vi "Get BLISS_Next Server or Done.vi"(7 "Queue in":refnum<queue>, 8 "error in":errorcluster, 11 "Data Parameters in":T1={"Server Index"=0, "username"="", "password"="", "Server Status List"=[{"Server Name"="BlissUT124", "connection\nsuccessful"=TRUE}, {"Server Name"="BlissMP146", "connection\nsuccessful"=TRUE}, {"Server Name"="BlissMP145", "connection\nsuccessful"=TRUE}, {"Server Name"="BlissMP140", "connection\nsuccessful"=TRUE}, {"Server Name"="BlissMP137", "connection\nsuccessful"=TRUE}, {"Server Name"="BlissMP135", "connection\nsuccessful"=TRUE}, {"Server Name"="BlissMP134", "connection\nsuccessful"=TRUE}, {"Server Name"="BlissMP132", "connection\nsuccessful"=TRUE}, {"Server Name"="BlissMA109", "connection\nsuccessful"=TRUE}, {"Server Name"="BlissMA107", "connection\nsuccessful"=TRUE}, {"Server Name"="BlissMA106", "connection\nsuccessful"=TRUE}, {"Server Name"="BlissMA101", "connection\nsuccessful"=TRUE}, {"Server Name"="BlissLU118", "connection\nsuccessful"=TRUE}, {"Server Name"="BlissLU117", "connection\nsuccessful"=TRUE}, {"Server Name"="BlissLU116", "connection\nsuccessful"=TRUE}, {"Server Name"="BlissLU115", "connection\nsuccessful"=TRUE}, {"Server Name"="BlissLU114", "connection\nsuccessful"=TRUE}, {"Server Name"="BlissLU113", "connection\nsuccessful"=TRUE}, {"Server Name"="BlissLU111", "connection\nsuccessful"=TRUE}, {"Server Name"="BlissLL185", "connection\nsuccessful"=TRUE}, {"Server Name"="BlissLL183", "connection\nsuccessful"=TRUE}, {"Server Name"="BlissLL173", "connection\nsuccessful"=TRUE}, {"Server Name"="BlissLL172", "connection\nsuccessful"=TRUE}, {"Server Name"="BlissLL171", "connection\nsuccessful"=TRUE}, {"Server Name"="BlissJH103", "connection\nsuccessful"=TRUE}, {"Server Name"="BlissJH102", "connection\nsuccessful"=TRUE}, {"Server Name"="BlissJH101", "connection\nsuccessful"=TRUE}, {"Server Name"="BlissJE116", "connection\nsuccessful"=TRUE}, {"Server Name"="BlissJE115", "connection\nsuccessful"=TRUE}, {"Server Name"="BlissJE114", "connection\nsuccessful"=TRUE}, {"Server Name"="BlissJE111", "connection\nsuccessful"=TRUE}, {"Server Name"="BlissHD183", "connection\nsuccessful"=TRUE}, {"Server Name"="BlissHD182", "connection\nsuccessful"=TRUE}, {"Server Name"="BlissHD181", "connection\nsuccessful"=TRUE}, {"Server Name"="BlissGPDFFPL", "connection\nsuccessful"=TRUE}, {"Server Name"="BlissEUWIPES", "connection\nsuccessful"=TRUE}, {"Server Name"="BlissEU179", "connection\nsuccessful"=TRUE}, {"Server Name"="BlissEU178", "connection\nsuccessful"=TRUE}, {"Server Name"="BlissEU177", "connection\nsuccessful"=TRUE}, {"Server Name"="Blissdvds02", "connection\nsuccessful"=TRUE}, {"Server Name"="BlissDOWIPES", "connection\nsuccessful"=TRUE}, {"Server Name"="BlissCR022", "connection\nsuccessful"=TRUE}, {"Server Name"="BlissCR021", "connection\nsuccessful"=TRUE}, {"Server Name"="BlissCG167", "connection\nsuccessful"=TRUE}, {"Server Name"="BlissCG166", "connection\nsuccessful"=TRUE}, {"Server Name"="BlissCG161", "connection\nsuccessful"=TRUE}, {"Server Name"="BlissCG160", "connection\nsuccessful"=TRUE}, {"Server Name"="BlissCG159", "connection\nsuccessful"=TRUE}, {"Server Name"="BlissCG158", "connection\nsuccessful"=TRUE}, {"Server Name"="BlissCG157", "connection\nsuccessful"=TRUE}, {"Server Name"="BlissCG156", "connection\nsuccessful"=TRUE}, {"Server Name"="BlissCG151", "connection\nsuccessful"=TRUE}, {"Server Name"="BlissCB172", "connection\nsuccessful"=TRUE}, {"Server Name"="BlissCB171", "connection\nsuccessful"=TRUE}, {"Server Name"="BlissCB108", "connection\nsuccessful"=TRUE}, {"Server Name"="BlissCB107", "connection\nsuccessful"=TRUE}, {"Server Name"="BlissBV181", "connection\nsuccessful"=TRUE}, {"Server Name"="BlissBV162", "connection\nsuccessful"=TRUE}, {"Server Name"="BlissAK177", "connection\nsuccessful"=TRUE}, {"Server Name"="BlissAK176", "connection\nsuccessful"=TRUE}, {"Server Name"="BlissAK175", "connection\nsuccessful"=TRUE}, {"Server Name"="BlissAK174", "connection\nsuccessful"=TRUE}, {"Server Name"="BlissAK173", "connection\nsuccessful"=TRUE}, {"Server Name"="BlissAK172", "connection\nsuccessful"=TRUE}, {"Server Name"="BlissAK171", "connection\nsuccessful"=TRUE}, {"Server Name"="BlissAK139", "connection\nsuccessful"=TRUE}, {"Server Name"="BlissAK134", "connection\nsuccessful"=TRUE}, {"Server Name"="BlissAK131", "connection\nsuccessful"=TRUE}, {"Server Name"="BlissAH163", "connection\nsuccessful"=TRUE}, {"Server Name"="BlissAH162", "connection\nsuccessful"=TRUE}, {"Server Name"="BlissAH161", "connection\nsuccessful"=TRUE}, {"Server Name"="BlissAH122", "connection\nsuccessful"=TRUE}, {"Server Name"="BlissAH121", "connection\nsuccessful"=TRUE}, {"Server Name"="BlissAD106", "connection\nsuccessful"=TRUE}, {"Server Name"="BlissAD104", "connection\nsuccessful"=TRUE}, {"Server Name"="BlissAB105", "connection\nsuccessful"=TRUE}, {"Server Name"="BlissAB104", "connection\nsuccessful"=TRUE}], "search criteria"={"views"="*.", "reject codes"="*.", "sizes"="*.", "BLISS Image Types"=enum."Get Both PBQA And Reject Images", "Start Timestamp"=timestamp(2145895200 s since 1904-01-01), "End Timesteamp"=timestamp(34618039200 s since 1904-01-01), "# Images per folder"=1, "Reset Filters Button"=FALSE}, "PBQA File List"=[], "Reject File List"=[], "Save to Folder"=path "", "Server List"=["BlissAB102", "BlissAB103", "BlissAB104", "BlissAB105", "BlissAD104", "BlissAD106", "BlissAH111", "BlissAH112", "BlissAH114", "BlissAH121", "BlissAH122", "BlissAH161", "BlissAH162", "BlissAH163", "BlissAK131", "BlissAK134", "BlissAK139", "BlissAK171", "BlissAK172", "BlissAK173", "BlissAK174", "BlissAK175", "BlissAK176", "BlissAK177", "BlissBH110", "BlissBV162", "BlissBV181", "BlissCB107", "BlissCB108", "BlissCB171", "BlissCB172", "BlissCG151", "BlissCG156", "BlissCG157", "BlissCG158", "BlissCG159", "BlissCG160", "BlissCG161", "BlissCG166", "BlissCG167", "BlissCR013", "BlissCR015", "BlissCR016", "BlissCR020", "BlissCR021", "BlissCR022", "BlissCR119", "BlissCRDev01", "BlissDOWIPES", "Blissdvds02", "BlissEU135D", "BlissEU177", "BlissEU178", "BlissEU179", "BlissEUDS001", "BlissEUWIPES", "BlissGPDFFPL", "BlissHD181", "BlissHD182", "BlissHD183", "BlissJE111", "BlissJE112", "BlissJE114", "BlissJE115", "BlissJE116", "BlissJH101", "BlissJH102", "BlissJH103", "BlissLL171", "BlissLL172", "BlissLL173", "BlissLL174", "BlissLL183", "BlissLL185", "BlissLS101", "BlissLS102", "BlissLU111", "BlissLU113", "BlissLU114", "BlissLU115", "BlissLU116", "BlissLU117", "BlissLU118", "BlissMA101", "BlissMA106", "BlissMA107", "BlissMA109", "BlissMP132", "BlissMP133", "BlissMP134", "BlissMP135", "BlissMP136", "BlissMP137", "BlissMP138", "BlissMP140", "BlissMP145", "BlissMP146", "BlissMP147", "BlissMR111", "BlissMR112", "BlissMR113", "BlissMX101", "BlissMX171", "BlissMX172", "BlissMX173", "BlissMX174", "BlissMX175", "BlissMX176", "BlissMX177", "BlissNK101", "BlissNK104", "BlissNK105", "BlissNK106", "BlissNK107", "BlissOC101", "BlissOC102", "BlissOC103", "BlissOC104", "BlissOC109", "BlissOC110", "BlissPESDXL", "BlissSI110", "BlissTR005", "BlissTR101", "BlissTR104", "BlissTR106", "BlissTR109", "BlissTR110", "BlissTR111", "BlissTR112", "BlissTR113", "BlissTR114", "BlissTR115", "BlissTR116", "BlissUT122", "BlissUT123", "BlissUT124", "BlissVP101", "BlissVP171"], "Start Time"=timestamp(3690155740.033191 s since 1904-01-01), "Use Line Subfolders"=FALSE, "Use View Subfolders"=FALSE} {"search criteria"."# Images per folder" min=1 max=10 step=1}) -> (0 "error out":errorcluster, 3 "Data Parameters out":T1={"Server Index"=138, "username"="varga.sm@pg.com", "password"="Magyar09", "Server Status List"=[{"Server Name"="BlissUT124", "connection\nsuccessful"=TRUE}, {"Server Name"="BlissMP146", "connection\nsuccessful"=TRUE}, {"Server Name"="BlissMP145", "connection\nsuccessful"=TRUE}, {"Server Name"="BlissMP140", "connection\nsuccessful"=TRUE}, {"Server Name"="BlissMP137", "connection\nsuccessful"=TRUE}, {"Server Name"="BlissMP135", "connection\nsuccessful"=TRUE}, {"Server Name"="BlissMP134", "connection\nsuccessful"=TRUE}, {"Server Name"="BlissMP132", "connection\nsuccessful"=TRUE}, {"Server Name"="BlissMA109", "connection\nsuccessful"=TRUE}, {"Server Name"="BlissMA107", "connection\nsuccessful"=TRUE}, {"Server Name"="BlissMA106", "connection\nsuccessful"=TRUE}, {"Server Name"="BlissMA101", "connection\nsuccessful"=TRUE}, {"Server Name"="BlissLU118", "connection\nsuccessful"=TRUE}, {"Server Name"="BlissLU117", "connection\nsuccessful"=TRUE}, {"Server Name"="BlissLU116", "connection\nsuccessful"=TRUE}, {"Server Name"="BlissLU115", "connection\nsuccessful"=TRUE}, {"Server Name"="BlissLU114", "connection\nsuccessful"=TRUE}, {"Server Name"="BlissLU113", "connection\nsuccessful"=TRUE}, {"Server Name"="BlissLU111", "connection\nsuccessful"=TRUE}, {"Server Name"="BlissLL185", "connection\nsuccessful"=TRUE}, {"Server Name"="BlissLL183", "connection\nsuccessful"=TRUE}, {"Server Name"="BlissLL173", "connection\nsuccessful"=TRUE}, {"Server Name"="BlissLL172", "connection\nsuccessful"=TRUE}, {"Server Name"="BlissLL171", "connection\nsuccessful"=TRUE}, {"Server Name"="BlissJH103", "connection\nsuccessful"=TRUE}, {"Server Name"="BlissJH102", "connection\nsuccessful"=TRUE}, {"Server Name"="BlissJH101", "connection\nsuccessful"=TRUE}, {"Server Name"="BlissJE116", "connection\nsuccessful"=TRUE}, {"Server Name"="BlissJE115", "connection\nsuccessful"=TRUE}, {"Server Name"="BlissJE114", "connection\nsuccessful"=TRUE}, {"Server Name"="BlissJE111", "connection\nsuccessful"=TRUE}, {"Server Name"="BlissHD183", "connection\nsuccessful"=TRUE}, {"Server Name"="BlissHD182", "connection\nsuccessful"=TRUE}, {"Server Name"="BlissHD181", "connection\nsuccessful"=TRUE}, {"Server Name"="BlissGPDFFPL", "connection\nsuccessful"=TRUE}, {"Server Name"="BlissEUWIPES", "connection\nsuccessful"=TRUE}, {"Server Name"="BlissEU179", "connection\nsuccessful"=TRUE}, {"Server Name"="BlissEU178", "connection\nsuccessful"=TRUE}, {"Server Name"="BlissEU177", "connection\nsuccessful"=TRUE}, {"Server Name"="Blissdvds02", "connection\nsuccessful"=TRUE}, {"Server Name"="BlissDOWIPES", "connection\nsuccessful"=TRUE}, {"Server Name"="BlissCR022", "connection\nsuccessful"=TRUE}, {"Server Name"="BlissCR021", "connection\nsuccessful"=TRUE}, {"Server Name"="BlissCG167", "connection\nsuccessful"=TRUE}, {"Server Name"="BlissCG166", "connection\nsuccessful"=TRUE}, {"Server Name"="BlissCG161", "connection\nsuccessful"=TRUE}, {"Server Name"="BlissCG160", "connection\nsuccessful"=TRUE}, {"Server Name"="BlissCG159", "connection\nsuccessful"=TRUE}, {"Server Name"="BlissCG158", "connection\nsuccessful"=TRUE}, {"Server Name"="BlissCG157", "connection\nsuccessful"=TRUE}, {"Server Name"="BlissCG156", "connection\nsuccessful"=TRUE}, {"Server Name"="BlissCG151", "connection\nsuccessful"=TRUE}, {"Server Name"="BlissCB172", "connection\nsuccessful"=TRUE}, {"Server Name"="BlissCB171", "connection\nsuccessful"=TRUE}, {"Server Name"="BlissCB108", "connection\nsuccessful"=TRUE}, {"Server Name"="BlissCB107", "connection\nsuccessful"=TRUE}, {"Server Name"="BlissBV181", "connection\nsuccessful"=TRUE}, {"Server Name"="BlissBV162", "connection\nsuccessful"=TRUE}, {"Server Name"="BlissAK177", "connection\nsuccessful"=TRUE}, {"Server Name"="BlissAK176", "connection\nsuccessful"=TRUE}, {"Server Name"="BlissAK175", "connection\nsuccessful"=TRUE}, {"Server Name"="BlissAK174", "connection\nsuccessful"=TRUE}, {"Server Name"="BlissAK173", "connection\nsuccessful"=TRUE}, {"Server Name"="BlissAK172", "connection\nsuccessful"=TRUE}, {"Server Name"="BlissAK171", "connection\nsuccessful"=TRUE}, {"Server Name"="BlissAK139", "connection\nsuccessful"=TRUE}, {"Server Name"="BlissAK134", "connection\nsuccessful"=TRUE}, {"Server Name"="BlissAK131", "connection\nsuccessful"=TRUE}, {"Server Name"="BlissAH163", "connection\nsuccessful"=TRUE}, {"Server Name"="BlissAH162", "connection\nsuccessful"=TRUE}, {"Server Name"="BlissAH161", "connection\nsuccessful"=TRUE}, {"Server Name"="BlissAH122", "connection\nsuccessful"=TRUE}, {"Server Name"="BlissAH121", "connection\nsuccessful"=TRUE}, {"Server Name"="BlissAD106", "connection\nsuccessful"=TRUE}, {"Server Name"="BlissAD104", "connection\nsuccessful"=TRUE}, {"Server Name"="BlissAB105", "connection\nsuccessful"=TRUE}, {"Server Name"="BlissAB104", "connection\nsuccessful"=TRUE}], "search criteria"={"views"="VISFE1,VISCC2", "reject codes"="R325,R326", "sizes"="S2,S3,S4,S5,S6,S7", "BLISS Image Types"=enum."Get Only Reject Images", "Start Timestamp"=timestamp(2145895200 s since 1904-01-01), "End Timesteamp"=timestamp(34618039200 s since 1904-01-01), "# Images per folder"=1, "Reset Filters Button"=FALSE}, "PBQA File List"=[], "Reject File List"=[], "Save to Folder"=path "D:/One Drive PG/Procter and Gamble/Varghese, Jacob - Deep Learning Vision System/Front Ear Foldover/BLISS Rejects (only R325 + R326) - not reviewed", "Server List"=["BlissAB102", "BlissAB103", "BlissAB104", "BlissAB105", "BlissAD104", "BlissAD106", "BlissAH111", "BlissAH112", "BlissAH114", "BlissAH121", "BlissAH122", "BlissAH161", "BlissAH162", "BlissAH163", "BlissAK131", "BlissAK134", "BlissAK139", "BlissAK171", "BlissAK172", "BlissAK173", "BlissAK174", "BlissAK175", "BlissAK176", "BlissAK177", "BlissBH110", "BlissBV162", "BlissBV181", "BlissCB107", "BlissCB108", "BlissCB171", "BlissCB172", "BlissCG151", "BlissCG156", "BlissCG157", "BlissCG158", "BlissCG159", "BlissCG160", "BlissCG161", "BlissCG166", "BlissCG167", "BlissCR013", "BlissCR015", "BlissCR016", "BlissCR020", "BlissCR021", "BlissCR022", "BlissCR119", "BlissCRDev01", "BlissDOWIPES", "Blissdvds02", "BlissEU135D", "BlissEU177", "BlissEU178", "BlissEU179", "BlissEUDS001", "BlissEUWIPES", "BlissGPDFFPL", "BlissHD181", "BlissHD182", "BlissHD183", "BlissJE111", "BlissJE112", "BlissJE114", "BlissJE115", "BlissJE116", "BlissJH101", "BlissJH102", "BlissJH103", "BlissLL171", "BlissLL172", "BlissLL173", "BlissLL174", "BlissLL183", "BlissLL185", "BlissLS101", "BlissLS102", "BlissLU111", "BlissLU113", "BlissLU114", "BlissLU115", "BlissLU116", "BlissLU117", "BlissLU118", "BlissMA101", "BlissMA106", "BlissMA107", "BlissMA109", "BlissMP132", "BlissMP133", "BlissMP134", "BlissMP135", "BlissMP136", "BlissMP137", "BlissMP138", "BlissMP140", "BlissMP145", "BlissMP146", "BlissMP147", "BlissMR111", "BlissMR112", "BlissMR113", "BlissMX101", "BlissMX171", "BlissMX172", "BlissMX173", "BlissMX174", "BlissMX175", "BlissMX176", "BlissMX177", "BlissNK101", "BlissNK104", "BlissNK105", "BlissNK106", "BlissNK107", "BlissOC101", "BlissOC102", "BlissOC103", "BlissOC104", "BlissOC109", "BlissOC110", "BlissPESDXL", "BlissSI110", "BlissTR005", "BlissTR101", "BlissTR104", "BlissTR106", "BlissTR109", "BlissTR110", "BlissTR111", "BlissTR112", "BlissTR113", "BlissTR114", "BlissTR115", "BlissTR116", "BlissUT122", "BlissUT123", "BlissUT124", "BlissVP101", "BlissVP171"], "Start Time"=timestamp(3690155740.033191 s since 1904-01-01), "Use Line Subfolders"=FALSE, "Use View Subfolders"=FALSE} {"search criteria"."# Images per folder" min=1 max=10 step=1})   [LabVIEW 2020]
uses:
  Get BLISS_Data Paramter Actions.ctl
  MC5e Gobal_Variables.vi
  Get BLISS_Global Command Q Control.ctl
  MC5e Squad_Info.ctl
  MC5e Unit_Status_List.ctl
  Get BLISS_Search Criteria.ctl
  MC5e Data_Parameters.ctl
panel:
  # "Reject codes only apply to rejects"
  # "Size filters only apply to PBQA folders"
  # "Reject codes only apply to rejects"
  # "Size filters only apply to PBQA folders"
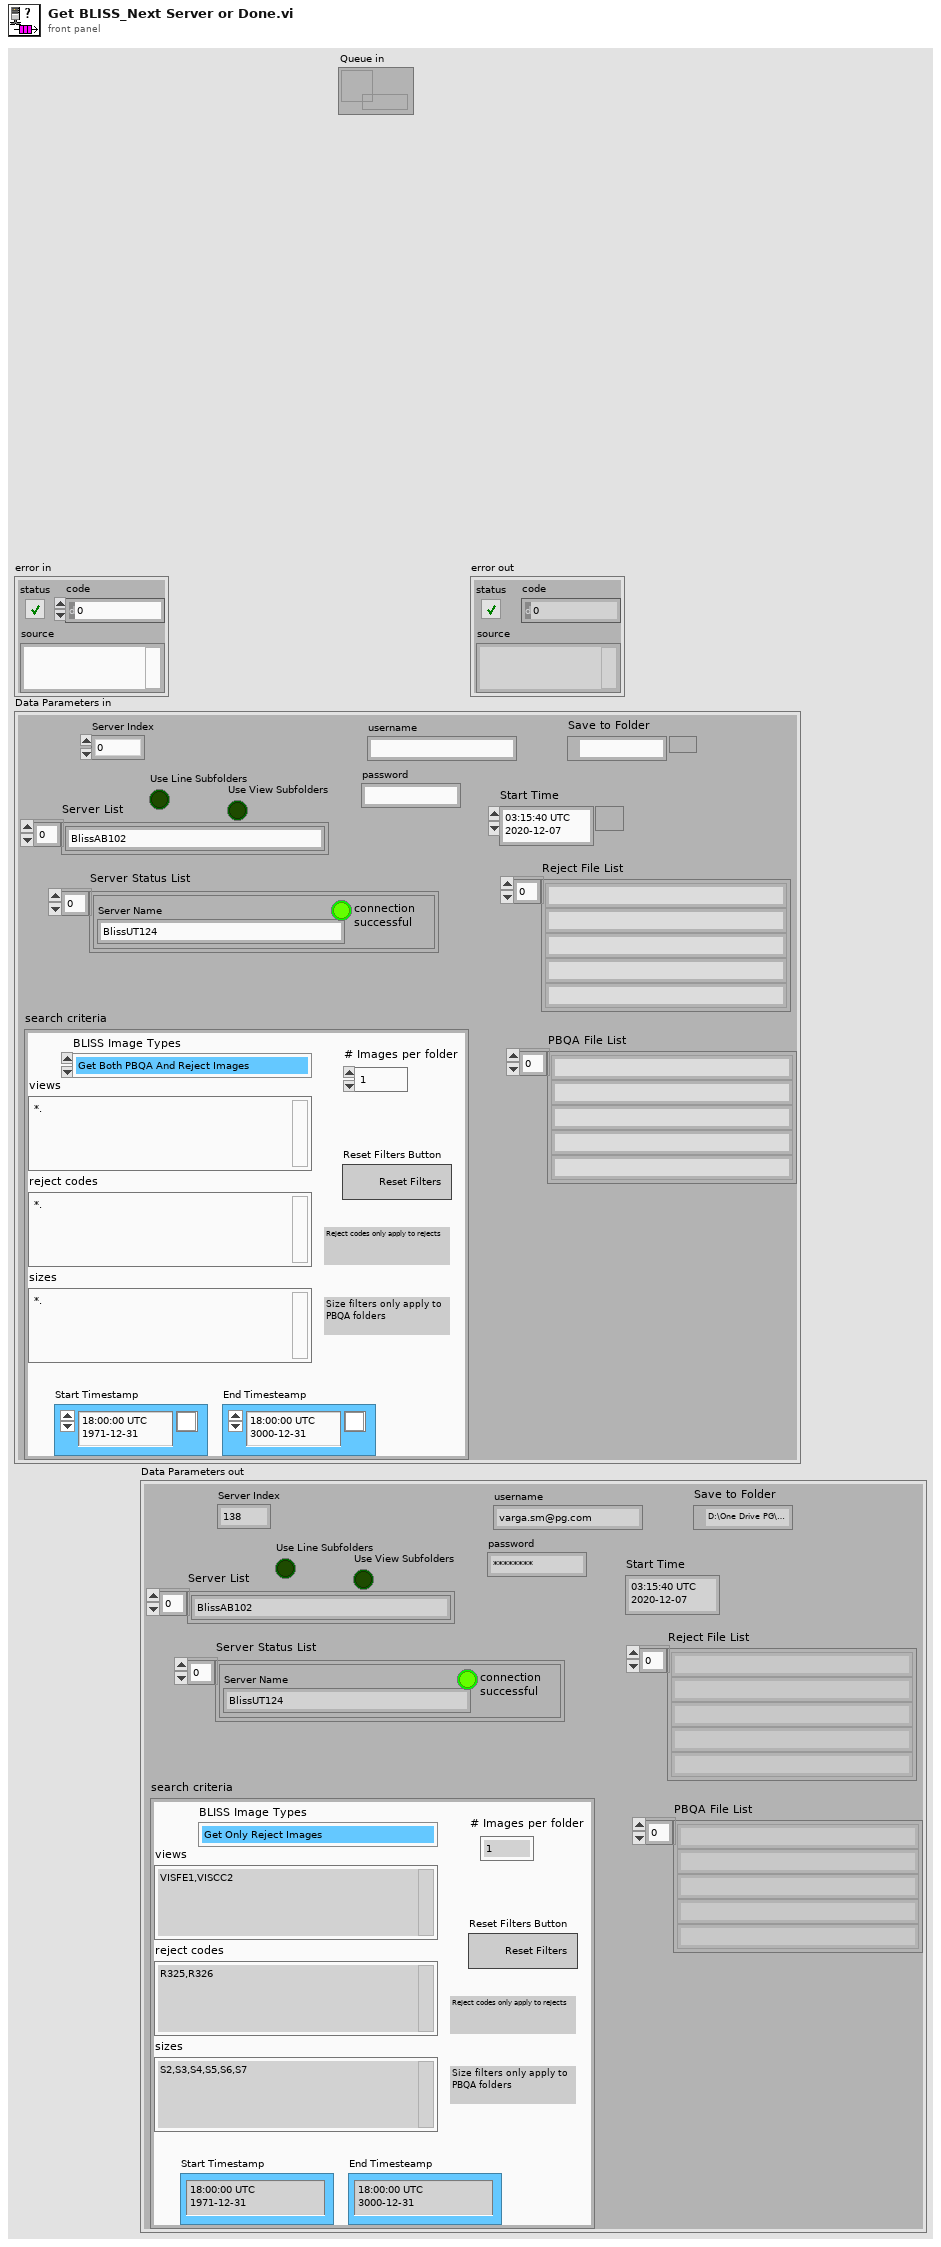
[diagram p1: front panel]
types:
  T1 = typedef "MC5e Data_Parameters.ctl" = cluster{"Server Index":i32, "username":string, "password":string, "Server Status List":T2, "search criteria":T4, "PBQA File List":string[], "Reject File List":string[], "Save to Folder":path, "Server List":string[], "Start Time":timestamp, "Use Line Subfolders":bool, "Use View Subfolders":bool}
  T2 = typedef "MC5e Unit_Status_List.ctl" = T3[]
  T3 = typedef "MC5e Unit_Status.ctl" = cluster{"Server Name":string, "connection\nsuccessful":bool}
  T4 = typedef "Get BLISS_Search Criteria.ctl" = cluster{"views":string, "reject codes":string, "sizes":string, "BLISS Image Types":enum16{"Get Only Reject Images", "Get Only PBQA Images", "Get Both PBQA And Reject Images"}, "Start Timestamp":timestamp, "End Timesteamp":timestamp, "# Images per folder":i32, "Reset Filters Button":bool}
  T5 = typedef "Get BLISS_Data Paramter Actions.ctl" = enum16{"Initialize", "Increment Index", "Reset Results", "Update", "Read"}
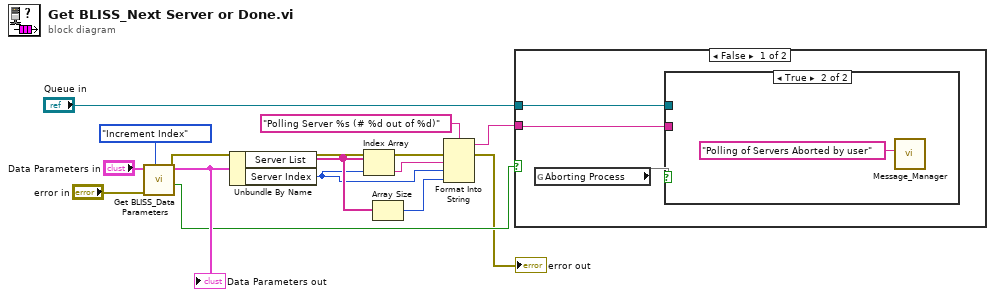
[diagram p0: block diagram]
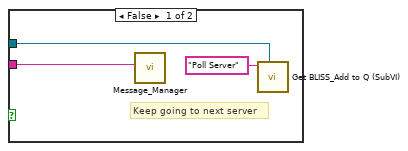
[diagram p2: hidden frame]
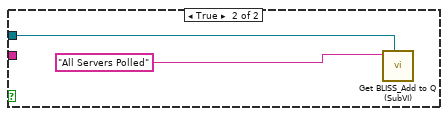
[diagram p3: hidden frame]
diagram:
  n1 = call "Get BLISS_Data Parameters.vi"("Data Action (Read)"=Get_BLISS_Data_Paramter_Actions."Increment Index", "error in"="error in", "Data Parameters in"="Data Parameters in") -> ("error out"=w3:errorcluster, "Rolled Over"=w5:bool, "Data Parameters out"=w7:T1)  [unwired: 6 in]
  "Data Parameters out" <- w7
  n2 = Unbundle By Name(w7) -> ("Server List"=w13:string[], "Server Index"=w12:i32)
  n3 = Index Array(array=w13, index=w12) -> (element=w8:string)
  n4 = Array Size(array=w13) -> (size(s)=w9:i32)
  n5 = Format Into String(format string="Polling Server %s (# %d out of %d)", error in=w3, w8, w12, w9) -> (resulting string=w11:string, error out=→"error out":errorcluster)  [unwired: 1 in]
  n6 = case shown="False" w5 {
    tunnel: "Queue in" -> [w17 w23]
    tunnel: w11 -> [w16 _]
    frame False {
      n7 = global read "MC5e Gobal_Variables.vi" "Aborting Process"() -> (w15)
      n8 = case shown="True" w15 {
        tunnel: w17 -> [w19 _]
        tunnel: w16 -> [w18 _]
        frame False {
          # "Keep going to next server"
          n9 = call "Message_Manager.vi"("New Entry"=w18) -> ()  [unwired: 5 in, 6 out]
          n10 = call "Get BLISS_Add to Q (SubVI).vi"("queue"=w19, "Command"="Poll Server") -> ()  [unwired: 9 in, 1 out]
        }
        frame True {
          n11 = call "Message_Manager.vi"("New Entry"="Polling of Servers Aborted by user") -> ()  [unwired: 5 in, 6 out]
        }
      }
    }
    frame True {
      n12 = call "Get BLISS_Add to Q (SubVI).vi"("queue"=w23, "Command"="All Servers Polled" ("Data")) -> ()  [unwired: 9 in, 1 out]
    }
  }
